vi "Tester_CSV_Parse_SVI.vi"(10 "Path to Tester CSV File":path, 11 "Catalog Number\nto search":string) -> (1 "Empty Row\nof Null Values":string[][](array[string]), 2 "Unformatted\nRow Data":string[](array[string]), 3 "All Catalog Numbers":string[](array[string]), 4 "Final 2D \nOutput Array":string[][](array[string]), 5 "Full Data":string[][](array[string]), 6 "Index of Searched \nCatalog Number":i32)   [LabVIEW 2021]
uses:
  <vilib>/Utility/file.llb/Read Delimited Spreadsheet (string).vi
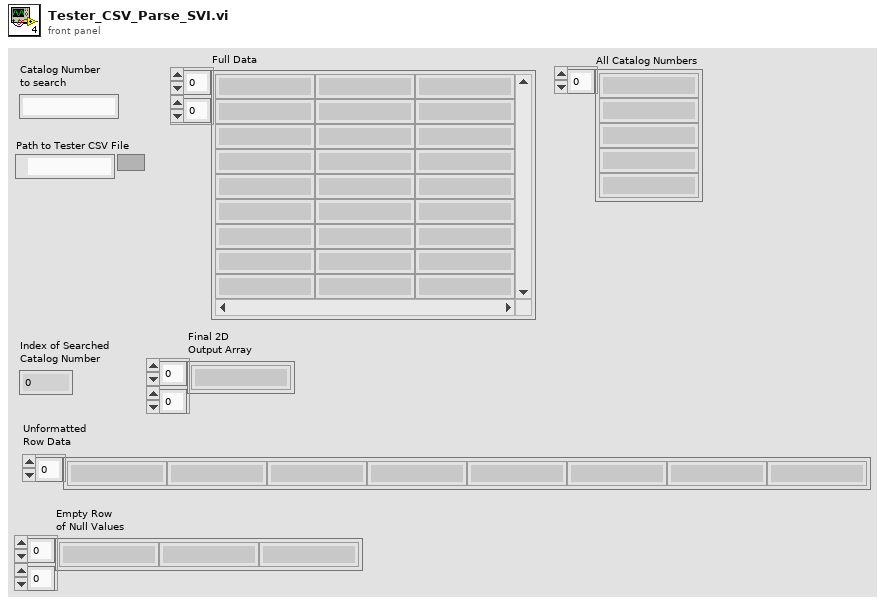
[diagram p1: front panel]
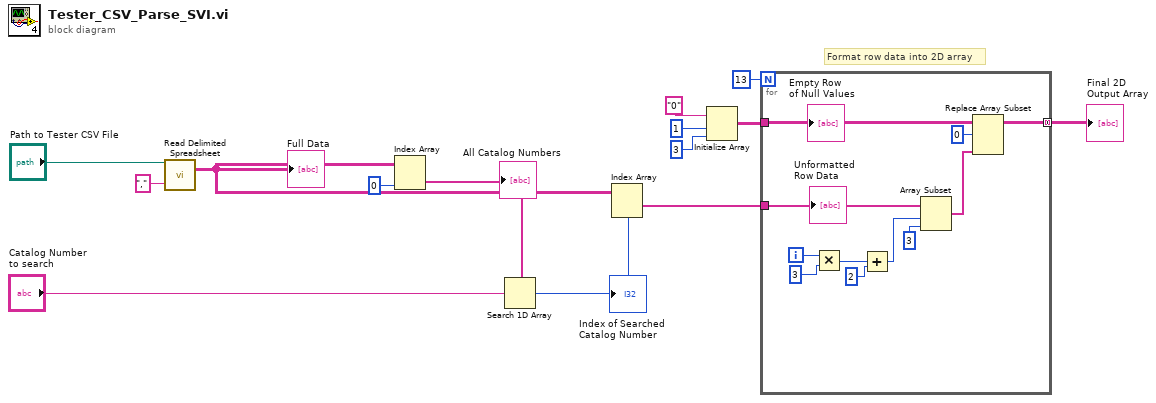
[diagram p0: block diagram]
diagram:
  # "Format row data into 2D array"
  n1 = call-poly <vilib>:"Read Delimited Spreadsheet.vi"("file path (dialog if empty)"="Path to Tester CSV File", "delimiter (\\t)"="," ("delimiter (\\t)")) -> ("all rows"=w6:string[][])  [unwired: 8 in, 5 out]
  "Full Data" <- w6
  n2 = Index Array(array=w6, index (col)=0 ("disabled index (col)")) -> (element=w4:string[])  [unwired: 1 in]
  "All Catalog Numbers" <- w4
  n3 = Search 1D Array(1D array=w4, element="Catalog Number\nto search") -> (index of element=w7:i32)  [unwired: 1 in]
  "Index of Searched \nCatalog Number" <- w7
  n4 = Index Array(array=w6, index (row)=w7) -> (element=w13:string[])  [unwired: 1 in]
  n5 = Initialize Array("0", 1 ("dimension size"), 3 ("dimension size")) -> (w12:string[][])
  n6 = for {
    N: 13 -> [_]
    tunnel: w12 -> [w20]
    tunnel: w13 -> [w21]
    tunnel: [w19] -> w14 mode=concatenating
    i -> [w15]
    n7 = Multiply(x=w15, y=3) -> (x*y=w24:i32)
    n8 = Add(x=w24, y=2) -> (x+y=w22:i32)
    n9 = Array Subset(array=w21, index=w22, length=3) -> (w18:string[])
    n10 = Replace Array Subset(array=w20, new element=w18, index (row)=0) -> (w19:string[][])  [unwired: 1 in]
    "Unformatted\nRow Data" <- w21
    "Empty Row\nof Null Values" <- w20
  }
  "Final 2D \nOutput Array" <- w14
